vi "ABR-Compute Cross-Correlation.vi"(0 "Neural (uV)":dbl[](array[numeric]), 5 "microphonic (uV)":dbl[](array[numeric]), 11 "error in (no error)":errorcluster) -> (4 "Corr Coef":dbl, 15 "error out":errorcluster)   [LabVIEW 2020]
uses:
  <vilib>/Analysis/baseanly.llb/Mean (DBL).vi
  <vilib>/Analysis/NI_AALBase.lvlib
  <vilib>/gmath/NI_Gmath.lvlib
panel:
  out "Graph":dbl[][](graph)
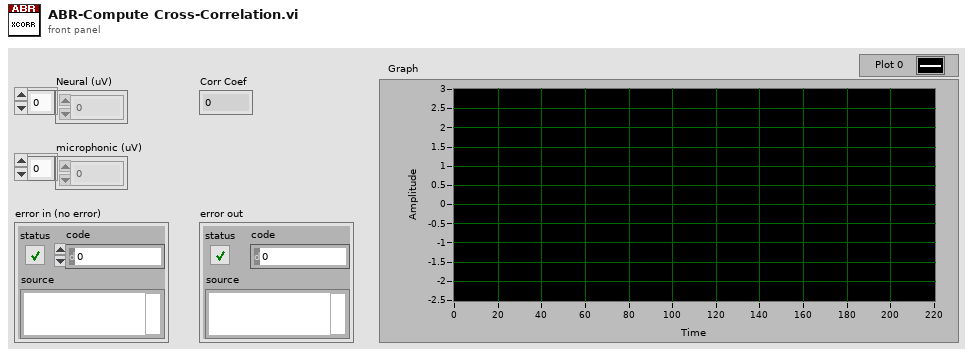
[diagram p1: front panel]
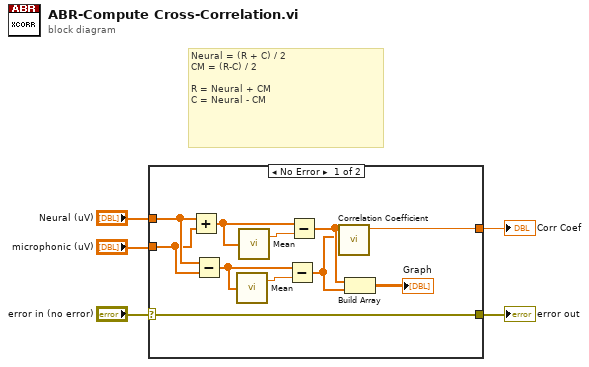
[diagram p0: block diagram]
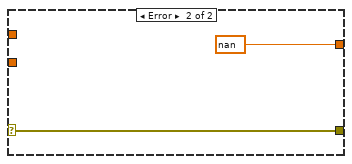
[diagram p2: hidden frame]
diagram:
  # "Neural = (R + C) / 2\nCM = (R-C) / 2\n\nR = Neural + CM\nC = Neural - CM"
  n1 = case shown="No Error" "error in (no error)" {
    selector: "error in (no error)" -> [w16 w17]
    tunnel: [w16 w17] -> w2
    tunnel: "Neural (uV)" -> [w15 _]
    tunnel: "microphonic (uV)" -> [w14 _]
    tunnel: [w9 nan ("correlation coefficient r")] -> w5
    frame No Error {
      n2 = Add(x=w15, y=w14) -> (x+y=w12:dbl[])
      n3 = Subtract(x=w15, y=w14) -> (x-y=w10:dbl[])
      n4 = call-poly <vilib>:"Mean.vi"("X"=w10) -> ("mean"=w11:dbl)  [unwired: 1 out]
      n5 = call-poly <vilib>:"Mean.vi"("X"=w12) -> ("mean"=w13:dbl)  [unwired: 1 out]
      n6 = Subtract(x=w10, y=w11) -> (x-y=w7:dbl[])
      n7 = Subtract(x=w12, y=w13) -> (x-y=w8:dbl[])
      n8 = call <vilib>:"Correlation Coefficient.vi"("Y"=w7, "X"=w8) -> ("correlation coefficient r"=w9:dbl)  [unwired: 8 in, 1 out]
      n9 = Build Array(w8, w7) -> (→"Graph":dbl[][])
    }
    frame Error {
    }
  }
  "Corr Coef" <- w5
  "error out" <- w2
